vi "calculateuncertaintyVer4.vi"(2 "Extinction ExtinctionUncertainity Size parameter and Number ofS sizes 2":T1={"Extinction"=[], "Extinction Uncertainty"=[], "Size parameters"=[], "Number ofSizes"=0.0, "GeometricCrossSection"=[], "Wave Length"=0.0, "SMPS Sizes"=[], "Concentration"=[], "Double Charge Correction"=FALSE, "Extincation Factor"=1.0, "Diameter Factor"=1.0, "Diameter Offset"=0.0, "Extinction Factor Flag"=FALSE, "Diameter Factor Flag"=FALSE, "Diameter Offset Flag"=FALSE, "Sizes"=[], "ExtinctionOrAbsorptionOrScattering"=0} {"ExtinctionOrAbsorptionOrScattering" scale=0.0..2.0}, 3 "refractive index, imaginary":dbl=0.10000000149011612 step=0.001 format="%.3f", 4 "refractive index, real":dbl=1.2999999523162842 step=0.001 format="%.3f") -> (0 "Uncertainty in Imaginary part":dbl format="%#_1g", 1 "Uncertainty in Real part":dbl format="%#_1g")   [LabVIEW 2013]
uses:
  BaesDataTypeDefinition.ctl
  <vilib>/Math Plots/3D Math Plots/3D Contour/3D Contour XCtrl/3D Contour.xctl
  <vilib>/gmath/NumericalOptimization/stopping criteria.ctl
  <vilib>/Analysis/1siggen.llb/Ramp Pattern by Samples.vi
  <vilib>/gmath/zero.llb/Newton Raphson Zero Finder (VI).vi
  <vilib>/gmath/NumericalOptimization/Downhill Simplex.vi
  <vilib>/Analysis/NI_AALBase.lvlib
  <vilib>/Math Plots/3D Math Plots/3D Contour/3D Contour Datatype/3D Contour Datatype.lvclass
  <vilib>/gmath/NI_Gmath.lvlib
  <vilib>/Math Plots/3D Math Plots/3D Contour/3D Contour Datatype/Public/Plot Helper (Vector).vi
  <vilib>/imath/engines/lvmath2/RunTimeEngine/Managers/WorkSpace/UID Generator.vi
  <vilib>/imath/engines/lvmath2/RunTimeEngine/BuiltInFunctions/contour/NIMS_contour(V, V).vi
  <vilib>/imathl/engines/lvmath/Functions/Error Handling/Create Error.vi
  <vilib>/imath/engines/lvmath2/RunTimeEngine/Managers/SymbolTable/Clear UID.vi
  <vilib>/imath/engines/lvmath2/RunTimeEngine/Managers/SymbolTable/NIMS_WorkSpace.lvlib
  <vilib>/imath/engines/lvmath2/RunTimeEngine/ErrorHandling/NIMS_Finalize Error.vi
panel:
  out "refractive index, imaginary 3":dbl
  out "refractive index, real 3":dbl
  out "refractive index, imaginary 2":dbl format="%#.3g"
  out "refractive index, real 2":dbl format="%#.3g"
  out "Array 3":dbl[](array[numeric])
  out "Array 2":dbl[](array[numeric]) format="%#.6g"
  out "Array":dbl[](array[numeric])
  out "Real Part MC":cluster{dbl[], dbl[]}(graph)
  in  "cluster":T2={"Imaginary or Real Part"=0.0, "Chi Square at Minimum"=0.0, "Extinction ExtinctionUncertainity Size parameter and Number ofS sizes"={"Extinction"=[], "Extinction Uncertainty"=[], "Size parameters"=[], "Number ofSizes"=0.0, "GeometricCrossSection"=[], "Wave Length"=0.0, "SMPS Sizes"=[], "Concentration"=[], "Double Charge Correction"=FALSE, "Extincation Factor"=1.0, "Diameter Factor"=1.0, "Diameter Offset"=0.0, "Extinction Factor Flag"=FALSE, "Diameter Factor Flag"=FALSE, "Diameter Offset Flag"=FALSE, "Sizes"=[], "ExtinctionOrAbsorptionOrScattering"=0}} {"Extinction ExtinctionUncertainity Size parameter and Number ofS sizes"."ExtinctionOrAbsorptionOrScattering" scale=0.0..2.0}
  out "Numeric 2":i32
  out "Numeric":i32
  out "3D Contour":refnum<class "3D Plot Datatype.lvclass">[](xcontrol)
  out "Chi Squared":dbl
  out "Chi Squared Imaginary":dbl[](array[numeric])=[1.7458156608733746, 2.259167774761544, 3.8146805575036473, 6.411304839763114, 10.047860655679122, 14.723114992903353, 20.436242940217376, 27.185713979953526, 34.970304890261, 43.78954822493611, 53.641277932357234]
  out "Ramp Pattern Imaginary":dbl[](array[numeric])=[0.1567711018030022, 0.1577711018030022, 0.1587711018030022, 0.1597711018030022, 0.1607711018030022, 0.1617711018030022, 0.1627711018030022, 0.1637711018030022, 0.1647711018030022, 0.1657711018030022, 0.1667711018030022]
  out "Chi Squared Real Part":dbl[](array[numeric])=[1.7458156608733746, 1.8138021473076842, 2.0074981029054553, 2.3266971611922957, 2.7715418766952578, 3.341681604102128, 4.037207690645187, 4.858019718358637, 5.804017563211861, 6.875028835060166, 8.070943802271257]
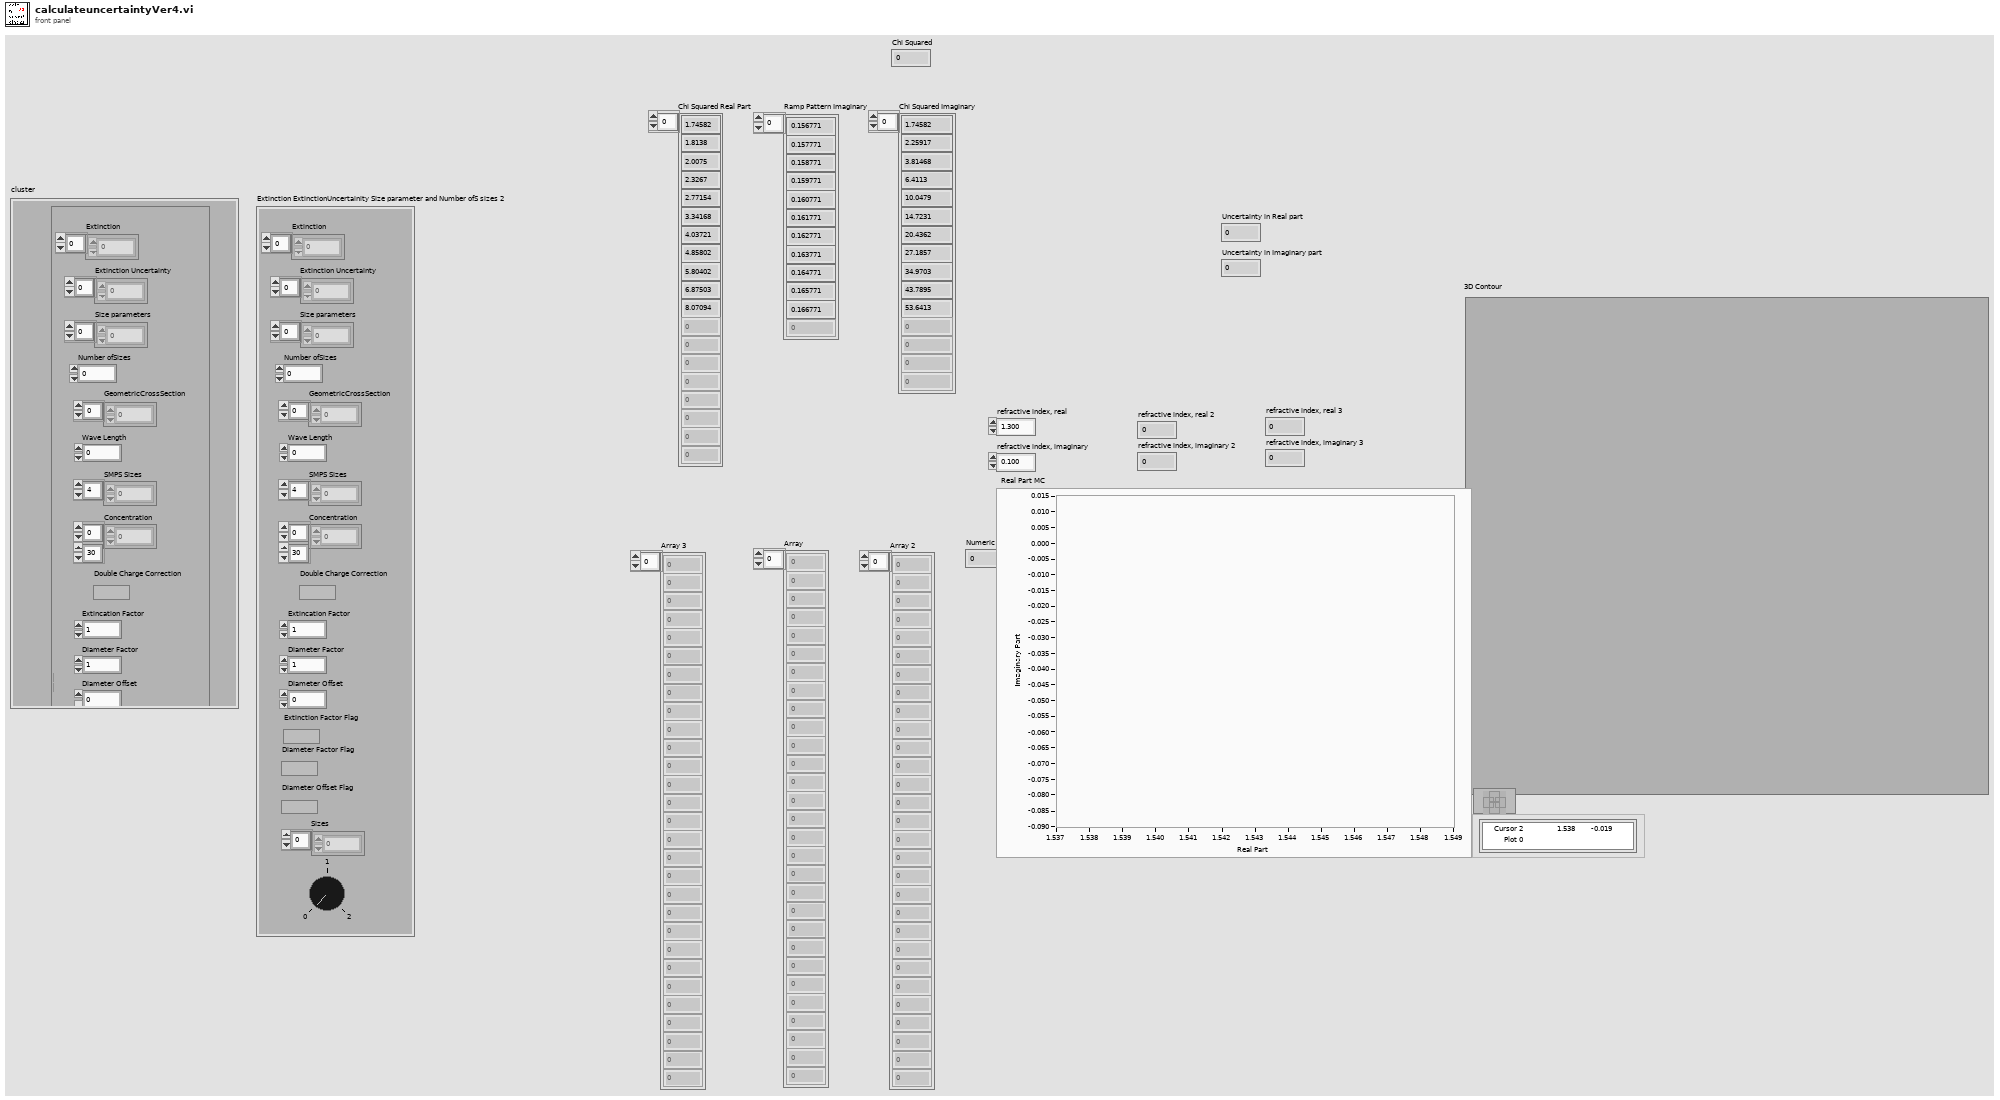
[diagram p1: front panel]
types:
  T1 = typedef "BaesDataTypeDefinition.ctl" = cluster{"Extinction":dbl[], "Extinction Uncertainty":dbl[], "Size parameters":dbl[], "Number ofSizes":dbl, "GeometricCrossSection":dbl[], "Wave Length":dbl, "SMPS Sizes":dbl[], "Concentration":dbl[][], "Double Charge Correction":bool, "Extincation Factor":dbl, "Diameter Factor":dbl, "Diameter Offset":dbl, "Extinction Factor Flag":bool, "Diameter Factor Flag":bool, "Diameter Offset Flag":bool, "Sizes":dbl[], "ExtinctionOrAbsorptionOrScattering":i8}
  T2 = cluster{"Imaginary or Real Part":dbl, "Chi Square at Minimum":dbl, "Extinction ExtinctionUncertainity Size parameter and Number ofS sizes":T1}
  T3 = typedef "NI_Gmath.lvlib/stopping criteria.ctl" = cluster{"function tolerance":dbl, "parameter tolerance":dbl, "max iterations":i32, "max function calls":i32, "gradient tolerance":dbl, "max time (sec)":dbl}
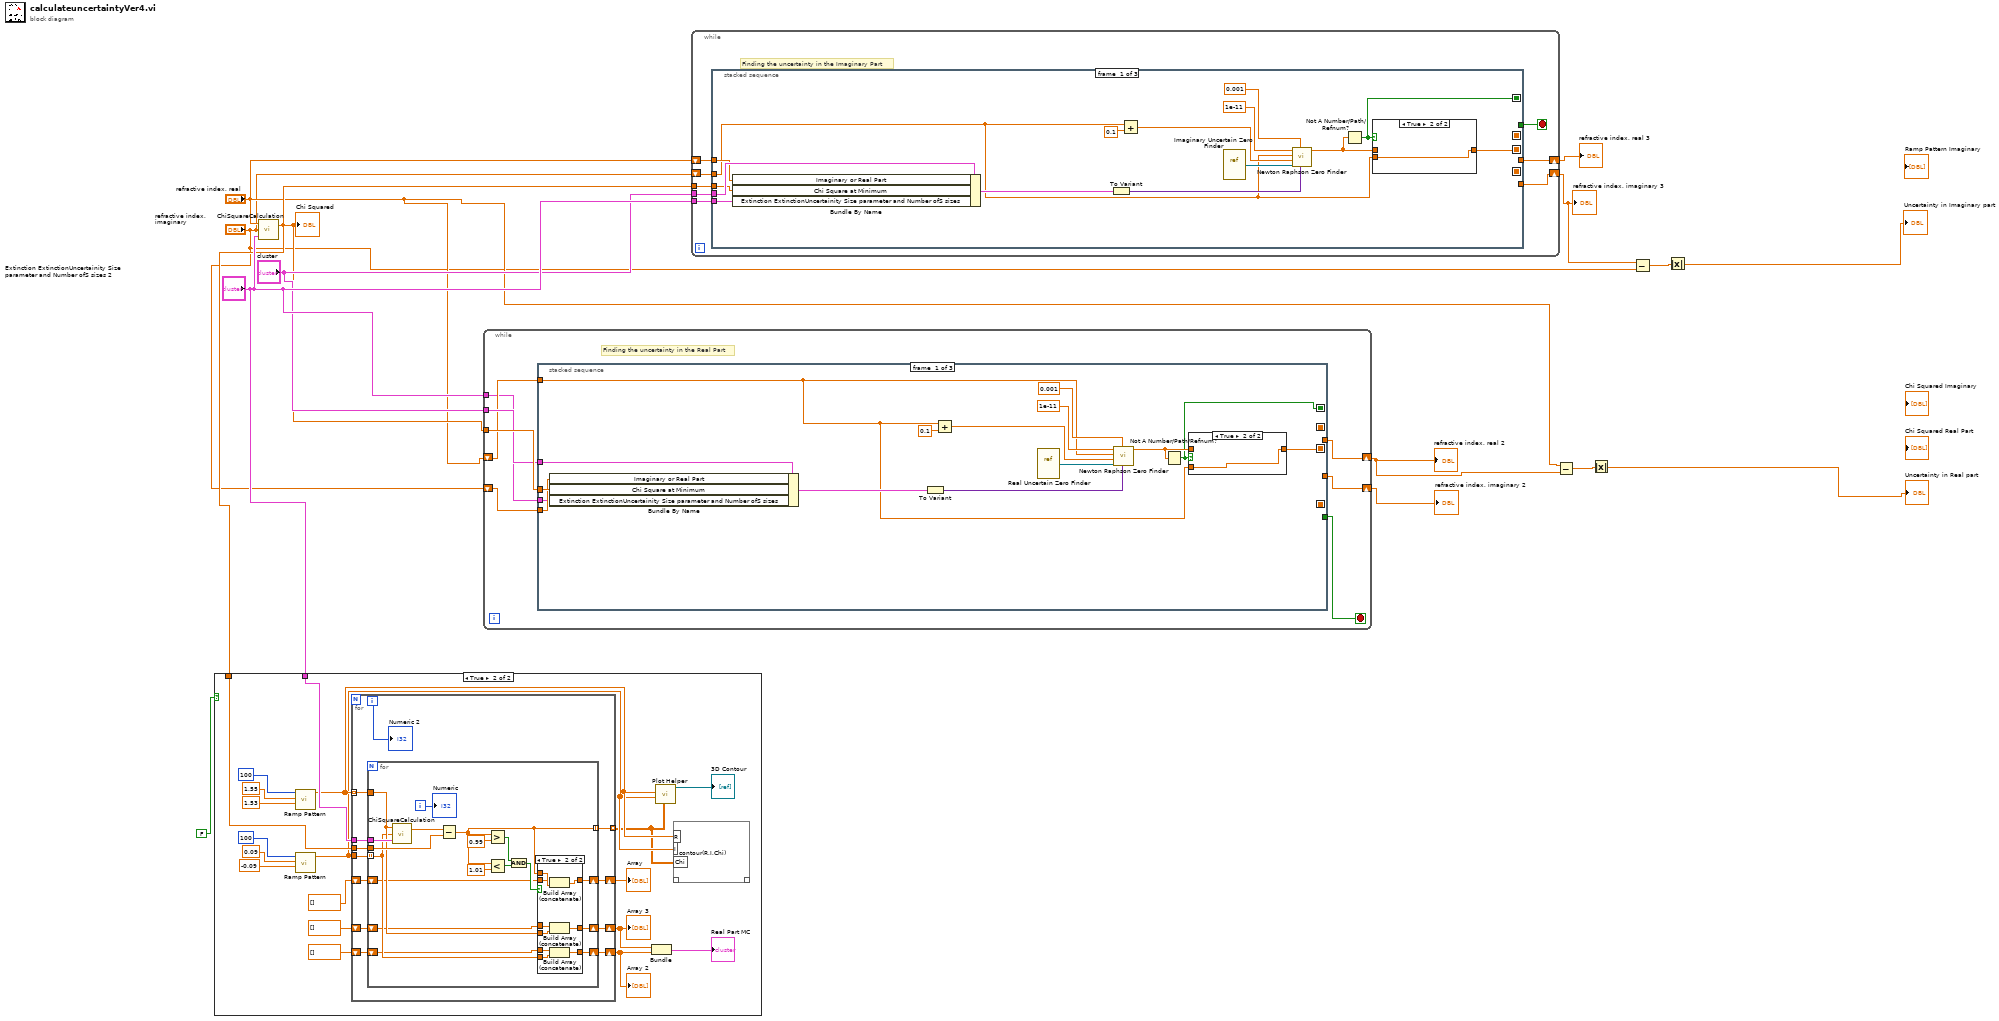
[diagram p0: block diagram]
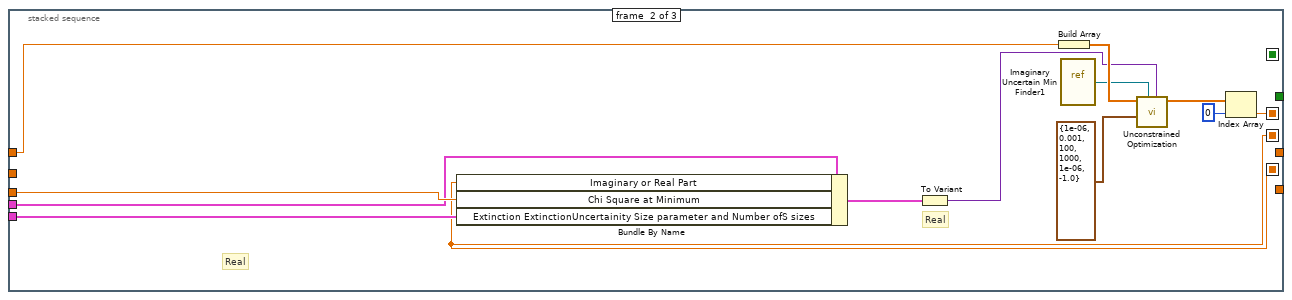
[diagram p3: hidden frame]
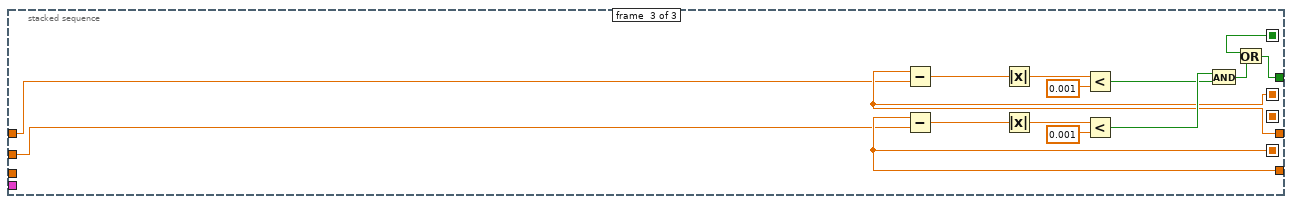
[diagram p4: hidden frame]
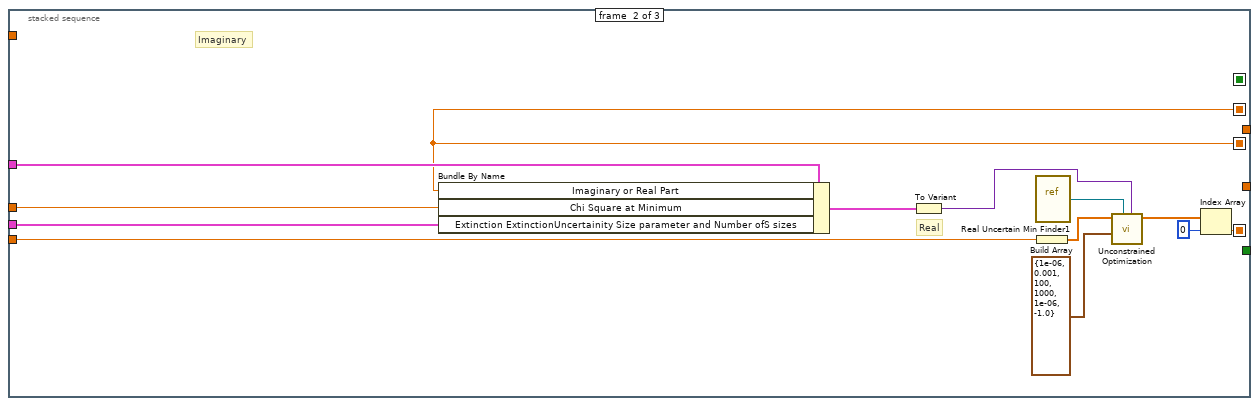
[diagram p6: hidden frame]
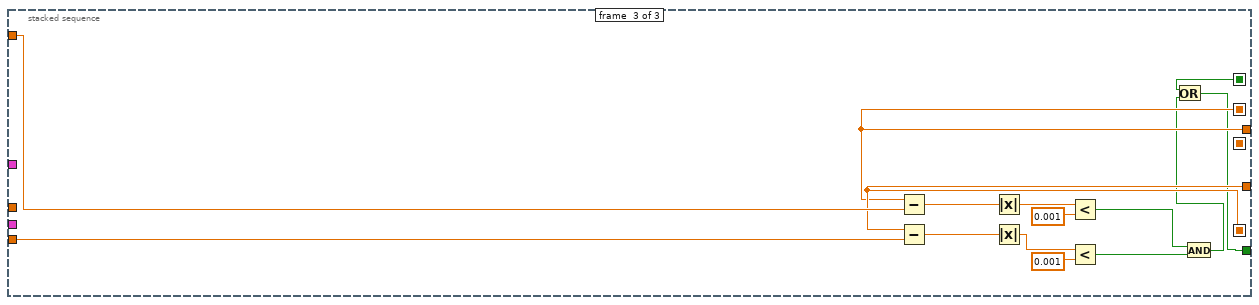
[diagram p7: hidden frame]
diagram:
  n1 = call "ChiSquareCalculation.vi"("Extinction ExtinctionUncertainity Size parameter and Number ofS sizes 2"="Extinction ExtinctionUncertainity Size parameter and Number ofS sizes 2", "refractive index, imaginary"="refractive index, imaginary", "refractive index, real"="refractive index, real") -> ("Chi Squared"=w10:dbl)  [unwired: 1 out]
  "Chi Squared" <- w10
  n2 = case shown="True" FALSE {
    tunnel: "Extinction ExtinctionUncertainity Size parameter and Number ofS sizes 2" -> [_ w27]
    tunnel: w10 -> [_ w25]
    frame False {
    }
    frame True {
      n3 = call-poly <vilib>:"Ramp Pattern.vi"("start"=1.53, "end"=1.55, "samples"=100) -> ("Ramp Pattern"=w17:dbl[])  [unwired: 7 in, 1 out]
      n4 = call-poly <vilib>:"Ramp Pattern.vi"("start"=-0.09, "end"=0.09, "samples"=100) -> ("Ramp Pattern"=w16:dbl[])  [unwired: 7 in, 1 out]
      n5 = for {
        tunnel: w17 -> [w87] mode=indexing
        tunnel: w16 -> [w86]
        tunnel: w27 -> [w85]
        tunnel: [w83] -> w15 mode=indexing
        tunnel: w25 -> [w82]
        shift-right: [w78] -> w19
        shift-left: dbl[] [] -> [w76]
        shift-right: [w77] -> w20
        shift-left: dbl[] [] -> [w79]
        shift-right: [w80] -> w18
        shift-left: dbl[] [] -> [w81]
        i -> [w84]
        n6 = for {
          tunnel: w87 -> [w96]
          tunnel: w86 -> [w95] mode=indexing
          tunnel: w85 -> [w105]
          tunnel: [w90] -> w83 mode=indexing
          tunnel: w82 -> [w103]
          shift-right: [w94] -> w80
          shift-left: w81 -> [w93]
          shift-right: [w92] -> w78
          shift-left: w76 -> [w91]
          shift-right: [w89] -> w77
          shift-left: w79 -> [w88]
          i -> [w104]
          n7 = call "ChiSquareCalculation.vi"("Extinction ExtinctionUncertainity Size parameter and Number ofS sizes 2"=w105, "refractive index, imaginary"=w95, "refractive index, real"=w96) -> ("Chi Squared"=w102:dbl)  [unwired: 1 out]
          n8 = Subtract(x=w102, y=w103) -> (x-y=w90:dbl)
          n9 = Greater?(x=w90, y=0.99) -> (0:w100:bool)
          n10 = Less?(x=w90, y=1.01) -> (x < y?=w101:bool)
          n11 = And(x=w100, y=w101) -> (x .and. y?=w99:bool)
          n12 = case shown="True" w99 {
            tunnel: w96 -> [_ w117]
            tunnel: w95 -> [_ w116]
            tunnel: [w106 w115] -> w89
            tunnel: [w108 w114] -> w94
            tunnel: w93 -> [w108 w113]
            tunnel: w90 -> [_ w112]
            tunnel: [w107 w111] -> w92
            tunnel: w91 -> [w107 w110]
            tunnel: w88 -> [w106 w109]
            frame False {
            }
            frame True {
              n13 = Build Array (concatenate)(w110, w112) -> (w111:dbl[])
              n14 = Build Array (concatenate)(w109, w117) -> (w115:dbl[])
              n15 = Build Array (concatenate)(w113, w116) -> (w114:dbl[])
            }
          }
          "Numeric" <- w104
        }
        "Numeric 2" <- w84
      }
      "Array" <- w19
      "Array 2" <- w18
      "Array 3" <- w20
      n16 = Bundle(w20, w18) -> (→"Real Part MC":cluster{dbl[], dbl[]})  [unwired: 1 in]
      n17 = call-poly <vilib>:"Plot Helper.vi"("z matrix"=w15, "y vector"=w16, "x vector"=w17) -> ("3D Plot lvclass Array out"=→"3D Contour":refnum<class "3D Plot Datatype.lvclass">[])  [unwired: 3 in, 5 out]
      n18 = mathscript code="contour(R,I,Chi)"("R"=w17, "I"=w16, "Chi"=w15) -> ()  [unwired: 1 in, 1 out]
    }
  }
  n19 = while {
    tunnel: w10 -> [w125]
    shift-right: [w119] -> w7
    shift-left: "refractive index, real" -> [w123]
    tunnel: "cluster" -> [w124]
    shift-right: [w120] -> w13
    shift-left: "refractive index, imaginary" -> [w122]
    tunnel: "Extinction ExtinctionUncertainity Size parameter and Number ofS sizes 2" -> [w121]
    stop <- w118 stop-if-true
    # "Finding the uncertainty in the Real Part"
    n20 = stacked-sequence {
      seq-local: [w129 _ _] -> [_ w143 _]
      seq-local: [_ w144 _] -> [_ _ w160]
      seq-local: [_ w143 _] -> [_ _ w159]
      seq-local: [w126 _ _] -> [_ _ w158]
      tunnel: w125 -> [w139 w154 _]
      tunnel: w124 -> [w140 w153 _]
      tunnel: w123 -> [w127 _ w167]
      tunnel: w122 -> [w138 w149 w161]
      tunnel: w121 -> [w132 w155 _]
      tunnel: [_ _ w160] -> w120
      tunnel: [_ _ w159] -> w119
      tunnel: [_ _ w156] -> w118
      frame #0 {
        n21 = Bundle By Name(cluster=w140, "Imaginary or Real Part"=w138, "Chi Square at Minimum"=w139, "Extinction ExtinctionUncertainity Size parameter and Number ofS sizes"=w132) -> (w137:T2)
        n22 = To Variant(anything=w137) -> (Variant=w136:variant)
        n23 = Add(x=w127, y=0.1) -> (x+y=w134:dbl)
        n24 = vi-ref "Real Uncertain Zero Finder.vi"() -> (w133:refnum<vi>)
        n25 = call-poly <vilib>:"Newton Raphson Zero Finder.vi"("data"=w136, "accuracy"=0.001, "f(x)"=w133, "end"=w134, "start"=w127, "h"=1e-11) -> ("zero"=w128:dbl)  [unwired: 2 in, 3 out]
        n26 = Not A Number/Path/Refnum?(number/path/refnum=w128) -> (NaN/Path/Refnum?=w126:bool)
        n27 = case shown="True" w126 {
          tunnel: [w141 w142] -> w129
          tunnel: w128 -> [w141 _]
          tunnel: w127 -> [_ w142]
          frame False {
          }
          frame True {
          }
        }
      }
      frame #1 {
        # "Imaginary"
        # "Real"
        n28 = Bundle By Name(cluster=w153, "Imaginary or Real Part"=w143, "Chi Square at Minimum"=w154, "Extinction ExtinctionUncertainity Size parameter and Number ofS sizes"=w155) -> (w152:T2)
        n29 = To Variant(anything=w152) -> (Variant=w148:variant)
        n30 = vi-ref "Real Uncertain Min Finder1.vi"() -> (w147:refnum<vi>)
        n31 = Build Array(w149) -> (w151:dbl[])
        n32 = call-poly <vilib>:"Unconstrained Optimization.vi"("function data"=w148, "objective function"=w147, "stopping criteria"=T3 {"function tolerance"=1e-06, "parameter tolerance"=0.001, "max iterations"=100, "max function calls"=1000, "gradient tolerance"=1e-06, "max time (sec)"=-1.0}, "start"=w151) -> ("minimum"=w146:dbl[])  [unwired: 4 in, 3 out]
        n33 = Index Array(array=w146, index=0) -> (element=w144:dbl)
      }
      frame #2 {
        n34 = Subtract(x=w159, y=w167) -> (x-y=w170:dbl)
        n35 = Subtract(x=w160, y=w161) -> (x-y=w165:dbl)
        n36 = Absolute Value(x=w170) -> (abs(x)=w169:dbl)
        n37 = Absolute Value(x=w165) -> (abs(x)=w164:dbl)
        n38 = Less?(x=w169, y=0.001) -> (x < y?=w166:bool)
        n39 = Less?(x=w164, y=0.001) -> (x < y?=w162:bool)
        n40 = And(x=w166, y=w162) -> (x .and. y?=w157:bool)
        n41 = Or(x=w158, y=w157) -> (x .or. y?=w156:bool)
      }
    }
  }
  "refractive index, real 2" <- w7
  "refractive index, imaginary 2" <- w13
  n42 = while {
    tunnel: w10 -> [w178]
    shift-right: [w171] -> w9
    shift-left: "refractive index, real" -> [w176]
    tunnel: "cluster" -> [w177]
    shift-right: [w172] -> w3
    shift-left: "refractive index, imaginary" -> [w175]
    tunnel: "Extinction ExtinctionUncertainity Size parameter and Number ofS sizes 2" -> [w174]
    stop <- w173 stop-if-true
    # "Finding the uncertainty in the Imaginary Part"
    n43 = stacked-sequence {
      seq-local: [w181 _ _] -> [_ w197 _]
      seq-local: [_ w198 _] -> [_ _ w215]
      seq-local: [_ w197 _] -> [_ _ w214]
      seq-local: [w179 _ _] -> [_ _ w211]
      tunnel: w178 -> [w192 w207 _]
      tunnel: w177 -> [w193 w206 _]
      tunnel: w176 -> [w183 w196 w213]
      tunnel: w175 -> [w182 _ w212]
      tunnel: w174 -> [w186 w208 _]
      tunnel: [_ _ w215] -> w171
      tunnel: [_ _ w214] -> w172
      tunnel: [_ _ w209] -> w173
      frame #0 {
        n44 = Bundle By Name(cluster=w193, "Imaginary or Real Part"=w183, "Chi Square at Minimum"=w192, "Extinction ExtinctionUncertainity Size parameter and Number ofS sizes"=w186) -> (w191:T2)
        n45 = To Variant(anything=w191) -> (Variant=w190:variant)
        n46 = Add(x=w182, y=0.1) -> (x+y=w188:dbl)
        n47 = vi-ref "Imaginary Uncertain Zero Finder.vi"() -> (w187:refnum<vi>)
        n48 = call-poly <vilib>:"Newton Raphson Zero Finder.vi"("data"=w190, "accuracy"=0.001, "f(x)"=w187, "end"=w188, "start"=w182, "h"=1e-11) -> ("zero"=w180:dbl)  [unwired: 2 in, 3 out]
        n49 = Not A Number/Path/Refnum?(number/path/refnum=w180) -> (NaN/Path/Refnum?=w179:bool)
        n50 = case shown="True" w179 {
          tunnel: [w194 w195] -> w181
          tunnel: w182 -> [_ w195]
          tunnel: w180 -> [w194 _]
          frame False {
          }
          frame True {
          }
        }
      }
      frame #1 {
        # "Real"
        # "Real"
        n51 = Bundle By Name(cluster=w206, "Imaginary or Real Part"=w197, "Chi Square at Minimum"=w207, "Extinction ExtinctionUncertainity Size parameter and Number ofS sizes"=w208) -> (w205:T2)
        n52 = To Variant(anything=w205) -> (Variant=w202:variant)
        n53 = Build Array(w196) -> (w204:dbl[])
        n54 = vi-ref "Imaginary Uncertain Min Finder1.vi"() -> (w201:refnum<vi>)
        n55 = call-poly <vilib>:"Unconstrained Optimization.vi"("function data"=w202, "objective function"=w201, "stopping criteria"=T3 {"function tolerance"=1e-06, "parameter tolerance"=0.001, "max iterations"=100, "max function calls"=1000, "gradient tolerance"=1e-06, "max time (sec)"=-1.0}, "start"=w204) -> ("minimum"=w200:dbl[])  [unwired: 4 in, 3 out]
        n56 = Index Array(array=w200, index=0) -> (element=w198:dbl)
      }
      frame #2 {
        n57 = Subtract(x=w215, y=w213) -> (x-y=w219:dbl)
        n58 = Subtract(x=w214, y=w212) -> (x-y=w223:dbl)
        n59 = Absolute Value(x=w219) -> (abs(x)=w218:dbl)
        n60 = Absolute Value(x=w223) -> (abs(x)=w222:dbl)
        n61 = Less?(x=w218, y=0.001) -> (x < y?=w216:bool)
        n62 = Less?(x=w222, y=0.001) -> (x < y?=w220:bool)
        n63 = And(x=w220, y=w216) -> (x .and. y?=w210:bool)
        n64 = Or(x=w211, y=w210) -> (x .or. y?=w209:bool)
      }
    }
  }
  "refractive index, real 3" <- w9
  "refractive index, imaginary 3" <- w3
  n65 = Subtract(x="refractive index, real", y=w7) -> (x-y=w8:dbl)
  n66 = Absolute Value(x=w8) -> (abs(x)=→"Uncertainty in Real part":dbl)
  n67 = Subtract(x=w3, y="refractive index, imaginary") -> (x-y=w4:dbl)
  n68 = Absolute Value(x=w4) -> (abs(x)=→"Uncertainty in Imaginary part":dbl)
